vi "Test Pair Index.vi"() -> ()   [LabVIEW 2020]
panel:
  out "Index":i32
  in  "String":string
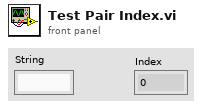
[diagram p1: front panel]
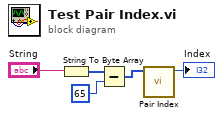
[diagram p0: block diagram]
diagram:
  n1 = String To Byte Array(string="String") -> (unsigned byte array=w4:u8[])
  n2 = Subtract(x=w4, y=u8 65) -> (x-y=w2:u8[])
  n3 = call "Pair Index.vi"("Pair"=w2) -> ("Index"=→"Index":i32)  [unwired: 10 in]
